vi "IP Address(Global).vi"() -> ()   [LabVIEW 2013]
panel:
  in  "IP Address":string
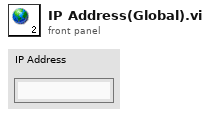
[diagram p1: front panel]
diagram:
